vi "Switches Demo.vi"() -> ()   [LabVIEW 2011]
panel:
  out "Boolean 8":bool
  in  "Boolean 7":bool
  out "Boolean 6":bool
  out "Boolean 5":bool
  out "Boolean 4":bool
  out "Boolean 3":bool
  out "Boolean 2":bool
  out "Boolean":bool
  in  "Latch untill released":bool
  in  "Latch when relased":bool
  in  "Latch when pressed":bool
  in  "Switch untill released":bool
  in  "Switch when pressed":bool
  in  "Switch when released":bool
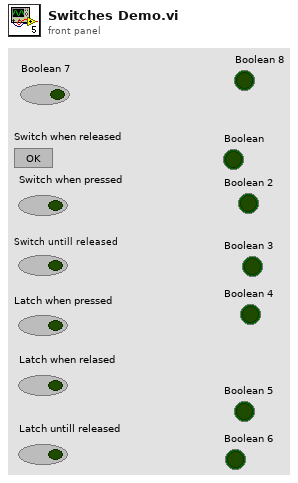
[diagram p1: front panel]
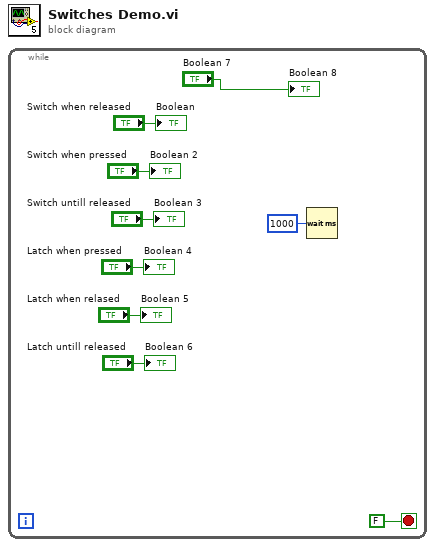
[diagram p0: block diagram]
diagram:
  n1 = while {
    stop <- FALSE stop-if-true
    n2 = Wait (ms)(milliseconds to wait=u32 1000) -> ()  [unwired: 1 out]
    "Boolean" <- "Switch when released"
    "Boolean 2" <- "Switch when pressed"
    "Boolean 3" <- "Switch untill released"
    "Boolean 4" <- "Latch when pressed"
    "Boolean 5" <- "Latch when relased"
    "Boolean 6" <- "Latch untill released"
    "Boolean 8" <- "Boolean 7"
  }
